vi "Configure System Timer (To).vi"(7 "System Parameters":T1={"Sys Period"=0.1, "Sys Mode"=enum."Normal", "Sys Burst #"=10, "Sys DC On"=10, "Sys DC Off"=10, "Sys State"=TRUE, "Sys Gate"=TRUE, "Sys Trig Edge"=TRUE, "Sys Ext Mode"=enum."Disabled", "Sys Trig Lev"=2.5, "Sys Gate Lev "=2.5, "Sys Gate Mode"=enum."Disabled"} {"Sys Gate Lev" format="%.4p"; "Sys Trig Lev" format="%.4p"; "Sys Period" format="%.6p"}, 8 "error in (no error)":errorcluster, 11 "VISA resource name":refnum<visa-resource-name>) -> (0 "error out":errorcluster, 3 "VISA resource name out":refnum<visa-resource-name>)   [LabVIEW 2012]
doc: "This VI demonstrates how to use the \"All Sys Parameters.ctl\" and individual configuration functions to configure the system timer (To).\n\nThe parameters \"Burst #\", \"DC On\", \"DC Off\", and \"Level\", \"Gate Polarity\", \"Edge\" are only updated when operating in the corresponding mode."
uses:
  System Parameters.ctl
  Public/Configure/Configure Sys (To) Mode (Normal).vi
  Public/Configure/Configure Sys (To) Mode (Single Shot).vi
  Public/Configure/Configure Sys (To) Mode (Burst).vi
  Public/Configure/Configure Sys (To) Mode (Duty Cycle).vi
  Quantum Composers 9000 Series.lvlib
panel:
  # "The parameters  \"Burst #\", \"DC On\", \"DC Off\", and \"Level\", \"Gate Polarity\", \"Edge\" are only updated when operating in the corresponding mode."
  # "Input"
  # "Triggered"
  # "Gated"
  # "Mode"
  # "Burst"
  # "Duty\nCycle"
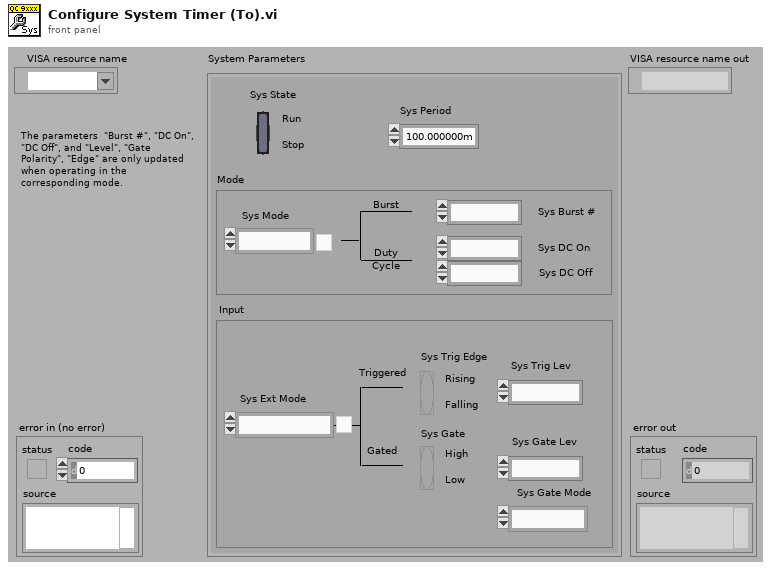
[diagram p1: front panel]
types:
  T1 = typedef "System Parameters.ctl" = cluster{"Sys Period":dbl, "Sys Mode":enum16{"Normal", "Single", "Burst", "Duty Cycle"}, "Sys Burst #":i32, "Sys DC On":i32, "Sys DC Off":i32, "Sys State":bool, "Sys Gate":bool, "Sys Trig Edge":bool, "Sys Ext Mode":enum16{"Disabled", "Triggered", "Gated", "Triggered & Gated"}, "Sys Trig Lev":dbl, "Sys Gate Lev ":dbl, "Sys Gate Mode":enum16{"Disabled", "Pulse Inhibit", "Output Inhibit", "Channel"}}
  T2 = enum16{"Normal", "Single", "Burst", "Duty Cycle"}
  T3 = enum16{"Disabled", "Triggered", "Gated", "Triggered & Gated"}
  T4 = enum16{"Disabled", "Pulse Inhibit", "Output Inhibit", "Channel"}
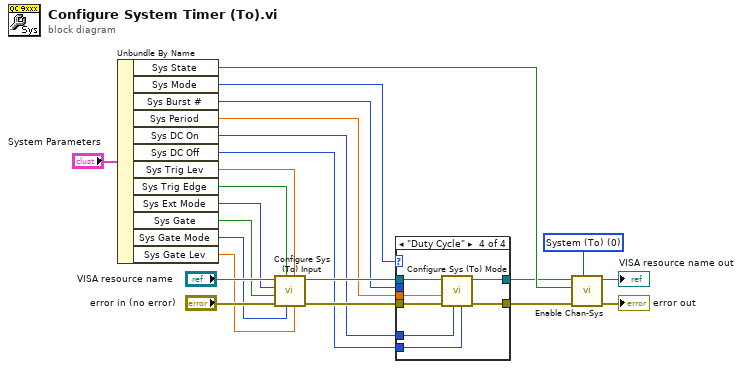
[diagram p0: block diagram]
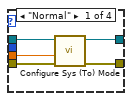
[diagram p2: hidden frame]
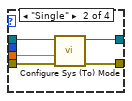
[diagram p3: hidden frame]
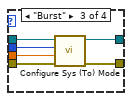
[diagram p4: hidden frame]
diagram:
  w19 = 0 items=["System (To)", "Channel A", "Channel B", "Channel C", "Channel D", "Channel E", "Channel F", "Channel G", "Channel H"] ("Channel (1:Chan A)")
  n1 = Unbundle By Name("System Parameters") -> ("Sys State"=w18:bool, "Sys Mode"=w11:T2, "Sys Burst #"=w9:i32, "Sys Period"=w10:dbl, "Sys DC On"=w8:i32, "Sys DC Off"=w7:i32, "Sys Trig Lev"=w5:dbl, "Sys Trig Edge"=w6:bool, "Sys Ext Mode"=w4:T3, "Sys Gate"=w3:bool, "Sys Gate Mode"=w2:T4, "Sys Gate Lev"=w1:dbl)
  n2 = call "Configure Sys (To) Input.vi"("Sys Gate Lev (2.5)"=w1, "Sys Trig Lev (2.5)"=w5, "Sys Gate Mode"=w2, "Sys Trig Edge (T: Rising)"=w6, "error in (no error)"="error in (no error)", "Sys Gate Logic (T:High)"=w3, "Sys Ext Mode"=w4, "VISA resource name"="VISA resource name") -> ("error out"=w14:errorcluster, "VISA resource name out"=w15:refnum<visa-resource-name>)  [unwired: 2 in]
  n3 = case shown="\"Duty Cycle\"" w11 {
    tunnel: [w27 w32 w38 w45] -> w13
    tunnel: [w26 w31 w37 w44] -> w12
    tunnel: w15 -> [w25 w30 w36 w43]
    tunnel: w14 -> [w24 w29 w35 w42]
    tunnel: w10 -> [w23 w28 w34 w41]
    tunnel: w9 -> [_ _ w33 _]
    tunnel: w8 -> [_ _ _ w40]
    tunnel: w7 -> [_ _ _ w39]
    frame "Normal" {
      n4 = call-poly "Configure Sys (To) Mode.vi"("error in (no error)"=w24, "Period (100 msec)"=w23, "VISA resource name"=w25) -> ("error out"=w26:errorcluster, "VISA resource name out"=w27:refnum<visa-resource-name>)  [unwired: 7 in]
    }
    frame "Single" {
      n5 = call-poly "Configure Sys (To) Mode.vi"("error in (no error)"=w29, "Period (100 msec)"=w28, "VISA resource name"=w30) -> ("error out"=w31:errorcluster, "VISA resource name out"=w32:refnum<visa-resource-name>)  [unwired: 7 in]
    }
    frame "Burst" {
      n6 = call-poly "Configure Sys (To) Mode.vi"("error in (no error)"=w35, "Period (100 msec)"=w34, "Burst # (10)"=w33, "VISA resource name"=w36) -> ("error out"=w37:errorcluster, "VISA resource name out"=w38:refnum<visa-resource-name>)  [unwired: 6 in]
    }
    frame "Duty Cycle" {
      n7 = call-poly "Configure Sys (To) Mode.vi"("DC Off (10)"=w39, "DC On (10)"=w40, "error in (no error)"=w42, "Period (100 msec)"=w41, "VISA resource name"=w43) -> ("error out"=w44:errorcluster, "VISA resource name out"=w45:refnum<visa-resource-name>)  [unwired: 5 in]
    }
  }
  n8 = call "Enable Chan-Sys.vi"("Channel (1:Chan A)"=w19, "error in (no error)"=w12, "State (T:Enabled)"=w18, "VISA resource name"=w13) -> ("error out"=→"error out":errorcluster, "VISA resource name out"=→"VISA resource name out":refnum<visa-resource-name>)  [unwired: 6 in]
